vi "ACQ Read.vi"(8 "error in (no error)":errorcluster, 11 "SimAsync in":refnum<class "SimAsync.lvclass">) -> (0 "error out":errorcluster, 3 "SimAsync out":refnum<class "SimAsync.lvclass">)   [LabVIEW 2014, in "SimAsync.lvlib" / "SimAsync.lvclass"]
uses:
  SimAsync.lvclass
  DriverMasterAsync/builds/DriverMasterAsync.lvlibp/Modules/HAL/DriverMasterAsync/DriverMasterAsyncClass/DriverMasterAsync.lvclass
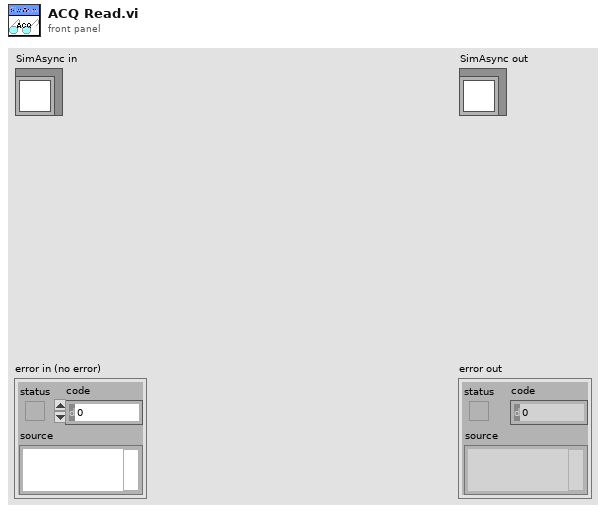
[diagram p1: front panel]
types:
  T1 = typedef "DriverMasterAsync.lvlibp/WINFAS 2 Data Queue.lvlib/Async Acquisition Data Cluster.ctl" = cluster{"Data":sgl[]}
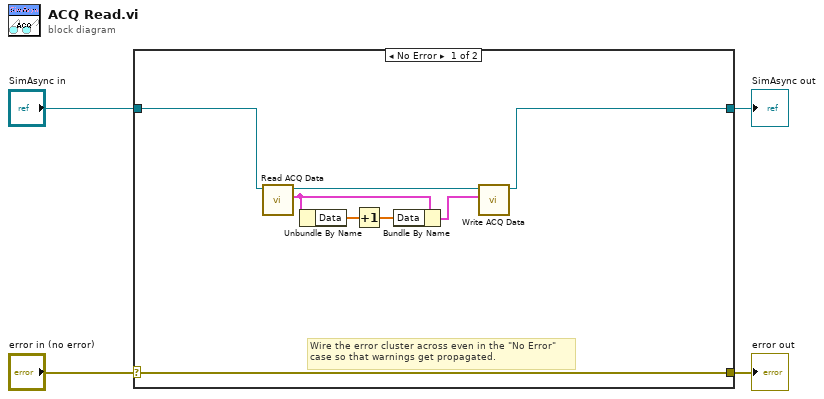
[diagram p0: block diagram]
diagram:
  n1 = case shown="No Error" "error in (no error)" {
    selector: "error in (no error)" -> [w12 w14]
    tunnel: [w12 w14] -> w3
    tunnel: [w9 w13] -> w1
    tunnel: "SimAsync in" -> [w11 w13]
    frame No Error {
      # "Wire the error cluster across even in the \"No Error\"\ncase so that warnings get propagated."
      n2 = call "Read ACQ Data.vi"("DriverMasterAsync in"=w11) -> ("ACQ Data"=w8:T1, "DriverMasterAsync out"=w10:refnum<class "SimAsync.lvclass">)  [unwired: 8 in, 1 out]
      n3 = Unbundle By Name(w8) -> ("Data"=w6:sgl[])
      n4 = Increment(x=w6) -> (x+1=w5:sgl[])
      n5 = Bundle By Name(cluster=w8, "Data"=w5) -> (w7:T1)
      n6 = call "Write ACQ Data.vi"("ACQ Data"=w7, "DriverMasterAsync in"=w10) -> ("DriverMasterAsync out"=w9:refnum<class "SimAsync.lvclass">)  [unwired: 8 in, 1 out]
    }
    frame Error {
    }
  }
  "error out" <- w3
  "SimAsync out" <- w1
